vi "Thermistor_Manual_Read.vi"(8 "error in":errorcluster, 9 "temp readings":T1, 11 "input cluster":T2={"Core"={"Current VI Reference"=refnum, "Close Panel on Exit?"=FALSE, "Exit"=FALSE, "Initialized?"=FALSE}, "Connections"={"cDAQ"={"Task"="", "Connected"=FALSE, "Active"=FALSE, "ID"=""}, "Camera"={"Session"="", "Connected"=FALSE, "Active"=FALSE, "Placeholder"=refnum}, "PSU"={"Port"="", "Connected"=FALSE, "Active"=FALSE}, "Arduino"={"Port"="", "Connected"=FALSE, "Active"=FALSE}}, "Data Acquisition"={"Setup"={"Label"="", "Operator"="", "Notes"="", "TempGrad"=1.0, "TargetTemp"=1.0, "Sample Volume"=1.0}, "Camera"={"Image"=refnum, "Save Image"=refnum, "Image Frequency"=20, "Rectangle"={"Left"=0, "Top"=0, "Right"=0, "Bottom"=0, "Rotation"=0.0}, "Calibration"={"Top Left"={"X"=0.0, "Y"=0.0}, "Top Right"={"X"=0.0, "Y"=0.0}, "Bottom Left"={"X"=0.0, "Y"=0.0}, "Bottom Right"={"X"=0.0, "Y"=0.0}, "Fixpoint"={"X"=0.0, "Y"=0.0}, "Scan Area"=0.0, "Fixpoint Area"=0.0, "Well Pixels"=[], "Valid"=FALSE}, "FocusPos"=0, "Display Mapping"=10}, "Thermistor"={"Sample Size"=1, "Calibration"={"B0.100"=[], "R25"=[], "c"=[], "State"=[], "V_S"=5.0, "R_S"=100.0}, "Timing Mode"=14713}, "Partition"={"Data"=[], "Cell Label"="", "Cell Color"=0, "Height"=10, "Width"=16, "Grid"=[]}, "Queue"={"Size"=1, "Queue"=refnum}, "Sample Rate"=1, "Active"=FALSE, "Ready"=FALSE, "Graph Mode"=0, "Gradient Buffer"=2}, "Control"={"Sample Rate"=1, "PID gains"={"proportional gain (Kc)"=1.0, "integral time (Ti, min)"=0.01, "derivative time (Td, min)"=0.0}}, "Manual Temp Control"={"TargetTemp"=1.0, "Mode"=0, "Active"=FALSE}} {"Manual Temp Control"."Mode" items=["Cool", "Heat"]; "Manual Temp Control"."TargetTemp" min=-40.0 max=40.0 step=0.5 format="%#_g °C"; "Control"."PID gains"."derivative time (Td, min)" format="%.3f"; "Control"."PID gains"."integral time (Ti, min)" format="%.3f"; "Control"."PID gains"."proportional gain (Kc)" format="%.3f"; "Control"."Sample Rate" min=1 max=20 step=1 format="%.0f Samples/sec"; "Data Acquisition"."Gradient Buffer" min=2 max=30 step=1; "Data Acquisition"."Graph Mode" items=["Thermistor Temperature", "Camera Temperature"]; "Data Acquisition"."Thermistor"."Timing Mode" items=["Automatic"=16097, "High Resolution"=10195, "High Speed"=14712, "Best 50 Hz Rejection"=14713, "Best 60 Hz Rejection"=14714, "Custom"=10137]; "Data Acquisition"."Thermistor"."Calibration"."R_S" min=0.1 max=1000.0 format="%#_g kOhm"; "Data Acquisition"."Thermistor"."Calibration"."V_S" min=5.0 max=48.0 format="%#_g V"; "Data Acquisition"."Thermistor"."Calibration"."R25" min=0.1 max=1000.0 format="%#_g kOhm"; "Data Acquisition"."Thermistor"."Calibration"."B0.100" min=100.0 max=10000.0 format="%#_g K"; "Data Acquisition"."Thermistor"."Sample Size" min=1 max=200; "Data Acquisition"."Sample Rate" min=20 max=240 format="%.0f samples/min"; "Data Acquisition"."Queue"."Size" min=1 max=200; "Data Acquisition"."Camera"."Display Mapping" items=["Default"=10, "Most Significant Bits"=11, "Full Dynamic"=12, "Downshift"=13, "Given Range"=14, "90% Dynamic"=15, "Given Percent Range"=16]; "Data Acquisition"."Camera"."Calibration"."Fixpoint"."Y" format="%.2f"; "Data Acquisition"."Camera"."Calibration"."Fixpoint"."X" format="%.2f"; "Data Acquisition"."Camera"."Calibration"."Top Left"."Y" format="%.2f"; "Data Acquisition"."Camera"."Calibration"."Top Left"."X" format="%.2f"; "Data Acquisition"."Camera"."Calibration"."Top Right"."Y" format="%.2f"; "Data Acquisition"."Camera"."Calibration"."Top Right"."X" format="%.2f"; "Data Acquisition"."Camera"."Calibration"."Bottom Left"."Y" format="%.2f"; "Data Acquisition"."Camera"."Calibration"."Bottom Left"."X" format="%.2f"; "Data Acquisition"."Camera"."Calibration"."Bottom Right"."Y" format="%.2f"; "Data Acquisition"."Camera"."Calibration"."Bottom Right"."X" format="%.2f"; "Data Acquisition"."Camera"."Rectangle"."Rotation" min=-90.0 max=90.0 step=1.0 format="%.2f"; "Data Acquisition"."Camera"."Rectangle"."Left" scale=0.0..1024.0; "Data Acquisition"."Camera"."Rectangle"."Right" scale=0.0..1024.0; "Data Acquisition"."Camera"."Image Frequency" min=1 max=60 step=1; "Data Acquisition"."Setup"."Sample Volume" min=0.0 max=500.0 format="%#_g µL"; "Data Acquisition"."Setup"."TargetTemp" min=-40.0 max=40.0 step=0.5 format="%#_g °C"; "Data Acquisition"."Setup"."TempGrad" min=-100.0 max=100.0 step=0.1 format="%#_g °C/min"}) -> (0 "error out":errorcluster, 3 "state":string)   [LabVIEW 2020]
uses:
  DataCluster.ctl
  <vilib>/userDefined/High Color/IMAQdx.ctl
  <vilib>/vision/Image Controls.llb/IMAQ Image.ctl
  <extravilib>/ChannelInstances/Tag-c(a[.](dbl),a[.](dbl))/))Channel.ctl
  <vilib>/Platform/TimedLoop/XDataNode/timing_clust.ctl
  <vilib>/Platform/TimedLoop/XDataNode/nitl_modes.ctl
  <vilib>/Platform/TimedLoop/XDataNode/wakeup.ctl
  <extravilib>/ChannelInstances/Tag-bool/Write With Abort.vi
  <extravilib>/ChannelInstances/Tag-c(a[.](dbl),a[.](dbl))/Read With Abort.vi
  <extravilib>/ChannelInstances/Tag-bool/Read With Abort.vi
  <extravilib>/ChannelInstances/Tag-bool/Instantiate.vi
  <extravilib>/ChannelInstances/Tag-c(a[.](dbl),a[.](dbl))/EndpointRead.vi
  <extravilib>/ChannelInstances/Tag-bool/EndpointRead.vi
  <extravilib>/ChannelInstances/Tag-bool/Endpoint.vi
  <vilib>/platform/TimedLoop/XDataNode/XDataNode.xnode
  <extravilib>/ChannelInstances/Tag-bool.lvlib
  <vilib>/Platform/TimedLoop/XDataNode/XDNodeRunTimeDep.lvlib
  <extravilib>/ChannelInstances/Tag-c(a[.](dbl),a[.](dbl)).lvlib
panel:
  out "Period (ms)":i64
  in  "Temp/Voltage":enum32{"Temp", "Voltage"}(radio)
  out "T8":dbl format="%.2f °C"
  out "T7":dbl format="%.2f °C"
  out "T6":dbl format="%.2f °C"
  out "T5":dbl format="%.2f °C"
  out "T4":dbl format="%.2f °C"
  out "T3":dbl format="%.2f °C"
  out "T2":dbl format="%.2f °C"
  out "T1":dbl format="%.2f °C"
  out "Status":string
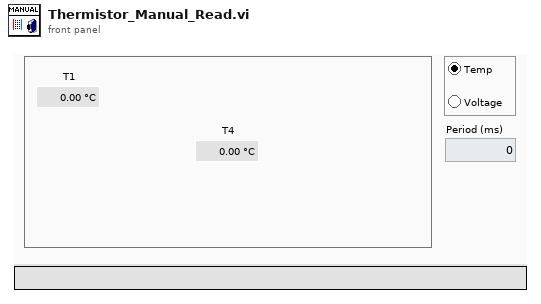
[diagram p1: front panel]
types:
  T1 = typedef "Tag-c(a[.](dbl),a[.](dbl)).lvlib/))Channel.ctl" = refnum<queue>
  T2 = typedef "DataCluster.ctl" = cluster{"Core":cluster{"Current VI Reference":refnum<vi>, "Close Panel on Exit?":bool, "Exit":bool, "Initialized?":bool}, "Connections":cluster{"cDAQ":cluster{"Task":refnum<k21>, "Connected":bool, "Active":bool, "ID":string}, "Camera":cluster{"Session":T3, "Connected":bool, "Active":bool, "Placeholder":T4}, "PSU":cluster{"Port":refnum<visa-resource-name>, "Connected":bool, "Active":bool}, "Arduino":cluster{"Port":refnum<visa-resource-name>, "Connected":bool, "Active":bool}}, "Data Acquisition":cluster{"Setup":cluster{"Label":string, "Operator":string, "Notes":string, "TempGrad":dbl, "TargetTemp":dbl, "Sample Volume":dbl}, "Camera":cluster{"Image":T4, "Save Image":T4, "Image Frequency":i32, "Rectangle":T5, "Calibration":cluster{"Top Left":T6, "Top Right":T6, "Bottom Left":T6, "Bottom Right":T6, "Fixpoint":T6, "Scan Area":dbl, "Fixpoint Area":dbl, "Well Pixels":cluster{"X":i32, "Y":i32}[][], "Valid":bool}, "FocusPos":u32, "Display Mapping":u32}, "Thermistor":cluster{"Sample Size":i32, "Calibration":cluster{"B0.100":dbl[], "R25":dbl[], "c":dbl[][], "State":bool[], "V_S":dbl, "R_S":dbl}, "Timing Mode":i32}, "Partition":cluster{"Data":string[][], "Cell Label":string, "Cell Color":u32, "Height":i32, "Width":i32, "Grid":string[][]}, "Queue":cluster{"Size":i32, "Queue":refnum<queue>}, "Sample Rate":i32, "Active":bool, "Ready":bool, "Graph Mode":u16, "Gradient Buffer":i32}, "Control":cluster{"Sample Rate":i32, "PID gains":cluster{"proportional gain (Kc)":dbl, "integral time (Ti, min)":dbl, "derivative time (Td, min)":dbl}}, "Manual Temp Control":cluster{"TargetTemp":dbl, "Mode":u16, "Active":bool}}
  T3 = typedef "IMAQdx.ctl" = refnum<k21>
  T4 = typedef "IMAQ Image.ctl" = refnum<image>
  T5 = typedef "IMAQ Rectangle" = cluster{"Left":i32, "Top":i32, "Right":i32, "Bottom":i32, "Rotation":dbl}
  T6 = typedef "IMAQ Point" = cluster{"X":sgl, "Y":sgl}
  T7 = typedef "Tag-bool.lvlib/))Channel.ctl" = refnum<queue>
  T8 = enum8{"Enabled", "Disabled", "Disabled and Grayed Out"}
  T9 = typedef "XDNodeRunTimeDep.lvlib/timing_clust.ctl" = cluster{"Expected End [f-1]":u64, "Actual End [f-1]":u64, "Finished Late? [f-1]":bool, "Expected End [i-1]":u64, "Actual End [i-1]":u64, "Finished Late? [i-1]":bool, "Expected Start [i]":u64, "Actual Start [i]":u64, "Expected Start [f]":u64, "Actual Start [f]":u64, "Source Name":string, "Structure Name":string, "Period":i64, "Deadline":i64, "Offset":i64, "Start":i64, "Priority":i32, "Timeout":i32, "Mode":T10, "Wakeup Reason":T11, "Error":errorcluster, "Source Type":string, "Secondary Source Type":string, "Global End Time":u64, "Global Start Time":u64, "Frame Duration":u64, "Iteration Duration":u64, "Assigned CPU":i32, "I/O Scan Engine Mode":u32}
  T10 = typedef "XDNodeRunTimeDep.lvlib/nitl_modes.ctl" = enum32{"No Change", "Process missed periods, maintain original phase", "Discard missed periods, maintain original phase", "Process missed periods, ignore original phase", "Discard missed periods, ignore original phase"}
  T11 = typedef "XDNodeRunTimeDep.lvlib/wakeup.ctl" = enum32{"Normal", "Aborted", "Asynchronous wakeup", "Timing source error", "Timed loop error", "Timeout"}
  T12 = cluster{"Temperature Readings Duplicate":dbl[], "Voltage Readings Duplicate":dbl[]}
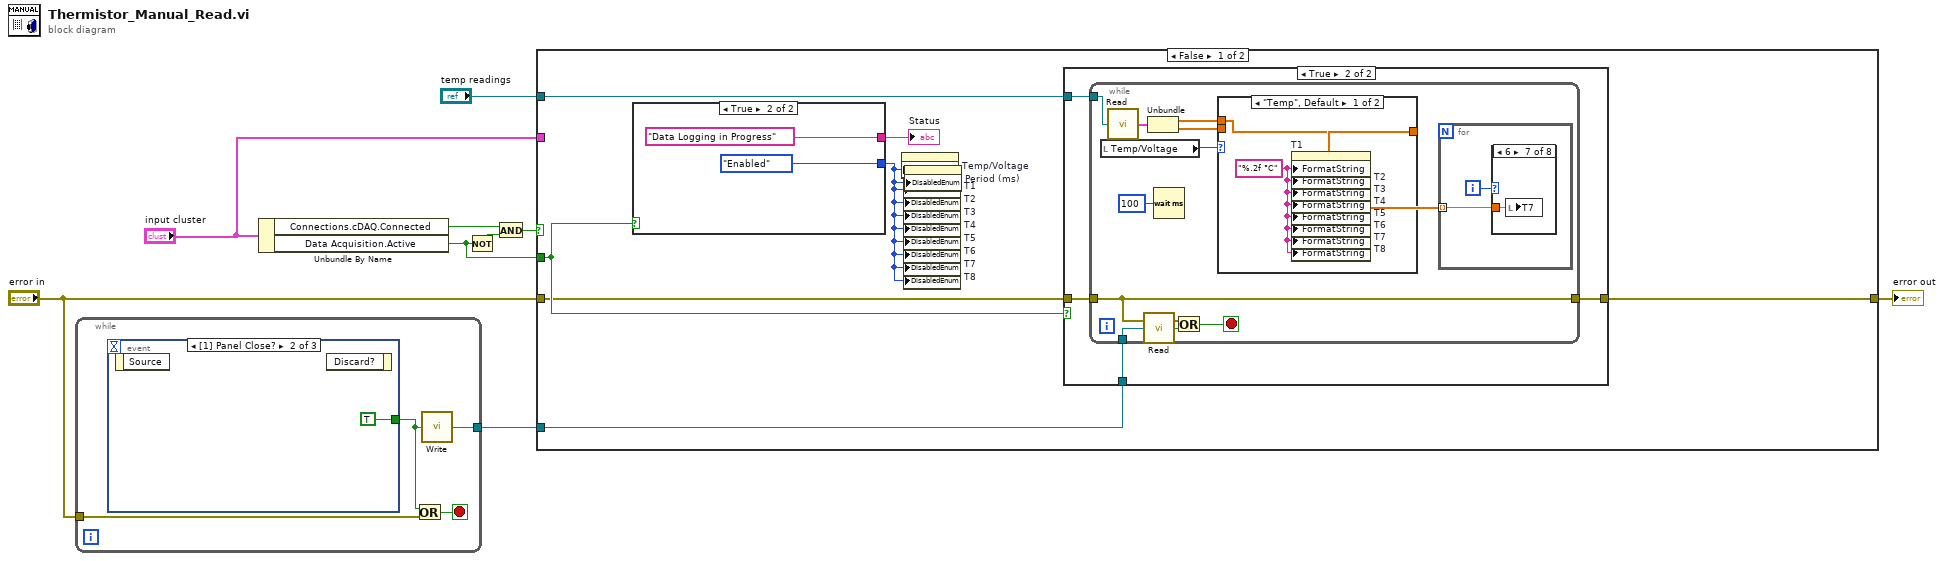
[diagram p0: block diagram]
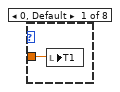
[diagram p3: hidden frame]
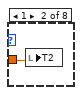
[diagram p4: hidden frame]
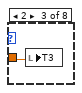
[diagram p5: hidden frame]
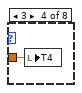
[diagram p6: hidden frame]
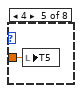
[diagram p7: hidden frame]
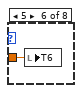
[diagram p8: hidden frame]
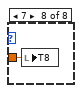
[diagram p9: hidden frame]
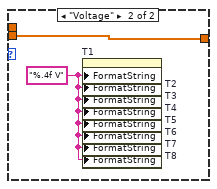
[diagram p10: hidden frame]
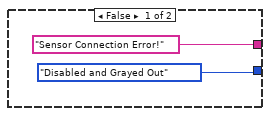
[diagram p11: hidden frame]
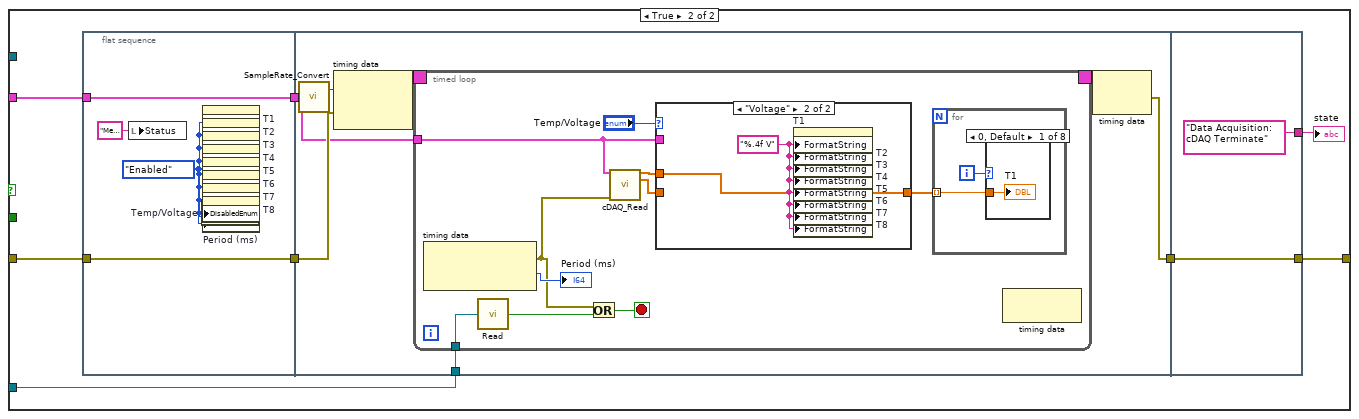
[diagram p12: hidden frame]
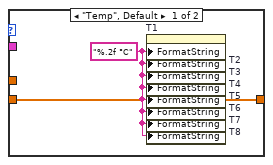
[diagram p13: hidden frame]
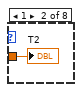
[diagram p14: hidden frame]
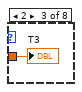
[diagram p15: hidden frame]
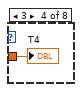
[diagram p16: hidden frame]
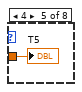
[diagram p17: hidden frame]
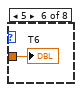
[diagram p18: hidden frame]
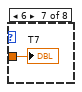
[diagram p19: hidden frame]
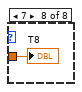
[diagram p20: hidden frame]
diagram:
  n1 = while {
    tunnel: "error in" -> [w11]
    tunnel: [w10] -> w6
    stop <- w12 stop-if-true
    n2 = event shown="[1] Panel Close?" {
      selector: _ -> [_ _ _]
      dyn-events: _ -> [_ _ _]
      timeout: _ -> [_ _ _]
      tunnel: [_ TRUE w18] -> w13
      event Timeout {
        n3 = event-data() -> ()  [unwired: 1 in, 1 out]
      }
      event Panel Close? {
        n4 = event-data() -> ()  [unwired: 1 in, 1 out]
        n5 = event-data() -> ()  [unwired: 2 in, 1 out]
      }
      event Key Up {
        # "Escape pressed?"
        n6 = event-data() -> ("ScanCode"=w17:i16)  [unwired: 1 in]
        n7 = Equal?(x=w17, y=i16 1) -> (x = y?=w15:bool)
        n8 = case shown="True" w15 {
          tunnel: [FALSE TRUE] -> w18
          frame False {
          }
          frame True {
          }
        }
      }
    }
    n9 = Or(x=w13, y=w11) -> (x .or. y?=w12:bool)
    n10 = call <extravilib>:"Write.vi"("element"=w13) -> ("channel"=w10:T7)  [unwired: 1 out]
  }
  n11 = Unbundle By Name("input cluster") -> ("Connections.cDAQ.Connected"=w9:bool, "Data Acquisition.Active"=w2:bool)
  n12 = Not(x=w2) -> (.not. x?=w3:bool)
  n13 = And(x=w9, y=w3) -> (x .and. y?=w4:bool)
  n14 = case shown="False" w4 {
    tunnel: "error in" -> [w24 w69]
    tunnel: [w21 w67] -> w8
    tunnel: w6 -> [w23 w65]
    tunnel: "input cluster" -> [_ w63]
    tunnel: w2 -> [w25 _]
    tunnel: "temp readings" -> [w22 _]
    frame False {
      n15 = case shown="True" w25 {
        tunnel: ["Sensor Connection Error!" ("String") "Data Logging in Progress" ("String")] -> w27
        tunnel: [T8."Disabled and Grayed Out" ("Disabled") T8."Enabled" ("Disabled")] -> w26
        frame False {
        }
        frame True {
        }
      }
      "Status" <- w27
      n16 = property on="Temp/Voltage" class="RadioBtnsControl (strict)"("DisabledEnum"=w26) -> ()  [unwired: 2 in, 2 out]
      n17 = property on="T1" class="DigNum (strict)"("DisabledEnum"=w26) -> ()  [unwired: 2 in, 2 out]
      n18 = property on="T2" class="DigNum (strict)"("DisabledEnum"=w26) -> ()  [unwired: 2 in, 2 out]
      n19 = property on="T3" class="DigNum (strict)"("DisabledEnum"=w26) -> ()  [unwired: 2 in, 2 out]
      n20 = property on="T4" class="DigNum (strict)"("DisabledEnum"=w26) -> ()  [unwired: 2 in, 2 out]
      n21 = property on="T5" class="DigNum (strict)"("DisabledEnum"=w26) -> ()  [unwired: 2 in, 2 out]
      n22 = property on="T6" class="DigNum (strict)"("DisabledEnum"=w26) -> ()  [unwired: 2 in, 2 out]
      n23 = property on="T7" class="DigNum (strict)"("DisabledEnum"=w26) -> ()  [unwired: 2 in, 2 out]
      n24 = property on="T8" class="DigNum (strict)"("DisabledEnum"=w26) -> ()  [unwired: 2 in, 2 out]
      n25 = property on="Period (ms)" class="DigNum (strict)"("DisabledEnum"=w26) -> ()  [unwired: 2 in, 2 out]
      n26 = case shown="True" w25 {
        tunnel: w24 -> [w28 w32]
        tunnel: w23 -> [_ w31]
        tunnel: w22 -> [_ w30]
        tunnel: [w28 w29] -> w21
        frame False {
        }
        frame True {
          n27 = while {
            tunnel: w32 -> [w37]
            tunnel: w31 -> [w43]
            tunnel: w30 -> [w40]
            tunnel: [w37] -> w29
            stop <- w41 stop-if-true
            n28 = local read "Temp/Voltage"() -> (w38:enum32{"Temp", "Voltage"})
            n29 = call <extravilib>:"Read.vi"("channel"=w40) -> ("element"=w39:T12)  [unwired: 1 in, 1 out]
            n30 = call <extravilib>:"Read.vi"("channel"=w43) -> ("element"=w42:bool)  [unwired: 1 in, 1 out]
            n31 = Unbundle(w39) -> ("Temperature Readings Duplicate"=w34:dbl[], "Voltage Readings Duplicate"=w35:dbl[])
            n32 = Wait (ms)(milliseconds to wait=u32 100) -> ()  [unwired: 1 out]
            n33 = Or(x=w37, y=w42) -> (x .or. y?=w41:bool)
            n34 = case shown="\"Temp\", Default" w38 {
              tunnel: [w54 w56] -> w36
              tunnel: w35 -> [_ w56]
              tunnel: w34 -> [w54 _]
              frame "Temp", Default {
                w55 = "%.2f °C"
                n35 = property on="T1" class="DigNum (strict)"("FormatString"=w55) -> ()  [unwired: 2 in, 2 out]
                n36 = property on="T2" class="DigNum (strict)"("FormatString"=w55) -> ()  [unwired: 2 in, 2 out]
                n37 = property on="T3" class="DigNum (strict)"("FormatString"=w55) -> ()  [unwired: 2 in, 2 out]
                n38 = property on="T4" class="DigNum (strict)"("FormatString"=w55) -> ()  [unwired: 2 in, 2 out]
                n39 = property on="T5" class="DigNum (strict)"("FormatString"=w55) -> ()  [unwired: 2 in, 2 out]
                n40 = property on="T6" class="DigNum (strict)"("FormatString"=w55) -> ()  [unwired: 2 in, 2 out]
                n41 = property on="T7" class="DigNum (strict)"("FormatString"=w55) -> ()  [unwired: 2 in, 2 out]
                n42 = property on="T8" class="DigNum (strict)"("FormatString"=w55) -> ()  [unwired: 2 in, 2 out]
              }
              frame "Voltage" {
                w57 = "%.4f V"
                n43 = property on="T1" class="DigNum (strict)"("FormatString"=w57) -> ()  [unwired: 2 in, 2 out]
                n44 = property on="T2" class="DigNum (strict)"("FormatString"=w57) -> ()  [unwired: 2 in, 2 out]
                n45 = property on="T3" class="DigNum (strict)"("FormatString"=w57) -> ()  [unwired: 2 in, 2 out]
                n46 = property on="T4" class="DigNum (strict)"("FormatString"=w57) -> ()  [unwired: 2 in, 2 out]
                n47 = property on="T5" class="DigNum (strict)"("FormatString"=w57) -> ()  [unwired: 2 in, 2 out]
                n48 = property on="T6" class="DigNum (strict)"("FormatString"=w57) -> ()  [unwired: 2 in, 2 out]
                n49 = property on="T7" class="DigNum (strict)"("FormatString"=w57) -> ()  [unwired: 2 in, 2 out]
                n50 = property on="T8" class="DigNum (strict)"("FormatString"=w57) -> ()  [unwired: 2 in, 2 out]
              }
            }
            n51 = for {
              tunnel: w36 -> [w44] mode=indexing
              i -> [w45]
              n52 = case shown="6" w45 {
                tunnel: w44 -> [w46 w47 w48 w49 w50 w51 w52 w53]
                frame 0, Default {
                  n53 = local write "T1"(w46) -> ()
                }
                frame 1 {
                  n54 = local write "T2"(w47) -> ()
                }
                frame 2 {
                  n55 = local write "T3"(w48) -> ()
                }
                frame 3 {
                  n56 = local write "T4"(w49) -> ()
                }
                frame 4 {
                  n57 = local write "T5"(w50) -> ()
                }
                frame 5 {
                  n58 = local write "T6"(w51) -> ()
                }
                frame 6 {
                  n59 = local write "T7"(w52) -> ()
                }
                frame 7 {
                  n60 = local write "T8"(w53) -> ()
                }
              }
            }
          }
        }
      }
    }
    frame True {
      n61 = flat-sequence {
        tunnel: w69 -> [w70]
        tunnel: [w70] -> w68
        tunnel: [w73] -> w64
        tunnel: w63 -> [w73]
        tunnel: w68 -> [w76]
        tunnel: [w75] -> w66
        tunnel: w65 -> [w80]
        tunnel: w64 -> [w74]
        tunnel: [w115] -> w67
        tunnel: w66 -> [w115]
        tunnel: ["Data Acquisition: cDAQ Terminate"] -> w62
        frame #0 {
          w71 = T8."Enabled" ("Disabled")
          n62 = local write "Status"("Measurement Active!" ("Status")) -> ()
          n63 = property on="Temp/Voltage" class="RadioBtnsControl (strict)"("DisabledEnum"=w71) -> ()  [unwired: 2 in, 2 out]
          n64 = property on="T1" class="DigNum (strict)"("DisabledEnum"=w71) -> ()  [unwired: 2 in, 2 out]
          n65 = property on="T2" class="DigNum (strict)"("DisabledEnum"=w71) -> ()  [unwired: 2 in, 2 out]
          n66 = property on="T3" class="DigNum (strict)"("DisabledEnum"=w71) -> ()  [unwired: 2 in, 2 out]
          n67 = property on="T4" class="DigNum (strict)"("DisabledEnum"=w71) -> ()  [unwired: 2 in, 2 out]
          n68 = property on="T5" class="DigNum (strict)"("DisabledEnum"=w71) -> ()  [unwired: 2 in, 2 out]
          n69 = property on="T6" class="DigNum (strict)"("DisabledEnum"=w71) -> ()  [unwired: 2 in, 2 out]
          n70 = property on="T7" class="DigNum (strict)"("DisabledEnum"=w71) -> ()  [unwired: 2 in, 2 out]
          n71 = property on="T8" class="DigNum (strict)"("DisabledEnum"=w71) -> ()  [unwired: 2 in, 2 out]
          n72 = property on="Period (ms)" class="DigNum (strict)"("DisabledEnum"=w71) -> ()  [unwired: 2 in, 2 out]
        }
        frame #1 {
          n73 = call "SampleRate_Convert.vi"("DataCluster"=w74) -> ("Sample dt (ms)"=w77:i64)  [unwired: 1 out]
          n74 = node-c288(w77, w76) -> (w79:T9)
          n75 = timed-loop {
            tunnel: w80 -> [w89]
            timing: w79 -> [_]
            timing-out: [_] -> w78
            tunnel: w74 -> [w84]
            stop <- w90 stop-if-true
            n76 = node-c288() -> (w81:errorcluster, →"Period (ms)":i64)  [unwired: 1 in]
            n77 = call <extravilib>:"Read.vi"("channel"=w89) -> ("element"=w88:bool)  [unwired: 1 in, 1 out]
            n78 = Or(x=w81, y=w88) -> (x .or. y?=w90:bool)
            n79 = call "cDAQ_Read.vi"("DataCluster"=w84, "error in"=w81) -> ("Voltage Readings"=w82:dbl[], "Temp Readings"=w83:dbl[])  [unwired: 6 in, 6 out]
            n80 = case shown="\"Voltage\"" "Temp/Voltage" {
              tunnel: w83 -> [w95 _]
              tunnel: [w95 w97] -> w86
              tunnel: w84 -> [_ _]
              tunnel: w82 -> [_ w97]
              frame "Temp", Default {
                w96 = "%.2f °C"
                n81 = property on="T1" class="DigNum (strict)"("FormatString"=w96) -> ()  [unwired: 2 in, 2 out]
                n82 = property on="T2" class="DigNum (strict)"("FormatString"=w96) -> ()  [unwired: 2 in, 2 out]
                n83 = property on="T3" class="DigNum (strict)"("FormatString"=w96) -> ()  [unwired: 2 in, 2 out]
                n84 = property on="T4" class="DigNum (strict)"("FormatString"=w96) -> ()  [unwired: 2 in, 2 out]
                n85 = property on="T5" class="DigNum (strict)"("FormatString"=w96) -> ()  [unwired: 2 in, 2 out]
                n86 = property on="T6" class="DigNum (strict)"("FormatString"=w96) -> ()  [unwired: 2 in, 2 out]
                n87 = property on="T7" class="DigNum (strict)"("FormatString"=w96) -> ()  [unwired: 2 in, 2 out]
                n88 = property on="T8" class="DigNum (strict)"("FormatString"=w96) -> ()  [unwired: 2 in, 2 out]
              }
              frame "Voltage" {
                w98 = "%.4f V"
                n89 = property on="T1" class="DigNum (strict)"("FormatString"=w98) -> ()  [unwired: 2 in, 2 out]
                n90 = property on="T2" class="DigNum (strict)"("FormatString"=w98) -> ()  [unwired: 2 in, 2 out]
                n91 = property on="T3" class="DigNum (strict)"("FormatString"=w98) -> ()  [unwired: 2 in, 2 out]
                n92 = property on="T4" class="DigNum (strict)"("FormatString"=w98) -> ()  [unwired: 2 in, 2 out]
                n93 = property on="T5" class="DigNum (strict)"("FormatString"=w98) -> ()  [unwired: 2 in, 2 out]
                n94 = property on="T6" class="DigNum (strict)"("FormatString"=w98) -> ()  [unwired: 2 in, 2 out]
                n95 = property on="T7" class="DigNum (strict)"("FormatString"=w98) -> ()  [unwired: 2 in, 2 out]
                n96 = property on="T8" class="DigNum (strict)"("FormatString"=w98) -> ()  [unwired: 2 in, 2 out]
              }
            }
            n97 = for {
              tunnel: w86 -> [w99] mode=indexing
              i -> [w100]
              n98 = case shown="0, Default" w100 {
                tunnel: w99 -> [w101 w102 w103 w104 w105 w106 w107 w108]
                frame 0, Default {
                  "T1" <- w101
                }
                frame 1 {
                  "T2" <- w102
                }
                frame 2 {
                  "T3" <- w103
                }
                frame 3 {
                  "T4" <- w104
                }
                frame 4 {
                  "T5" <- w105
                }
                frame 5 {
                  "T6" <- w106
                }
                frame 6 {
                  "T7" <- w107
                }
                frame 7 {
                  "T8" <- w108
                }
              }
            }
            n99 = node-c288() -> ()  [unwired: 1 in, 1 out]
          }
          n100 = node-c288(w78) -> (w75:errorcluster)
        }
        frame #2 {
        }
      }
      "state" <- w62
    }
  }
  "error out" <- w8
